vi "GetReferenceByUID_traverser.vi"(4 "context in":variant, 5 "objref":refnum<vi>) -> (1 "context out":variant, 2 "traverse flags":i32)   [LabVIEW 2013]
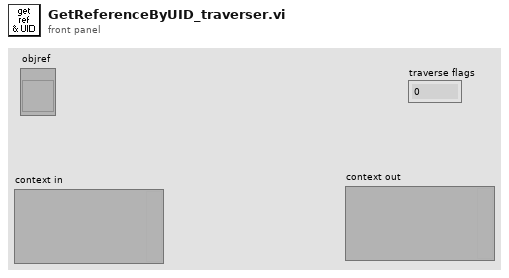
[diagram p1: front panel]
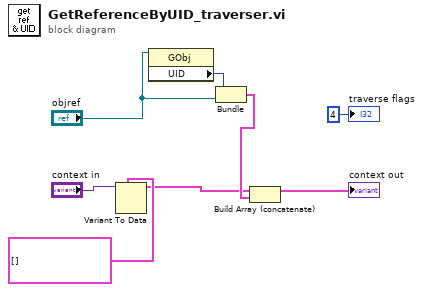
[diagram p0: block diagram]
diagram:
  n1 = Variant To Data(type=cluster{"UID":i32, "objref":refnum<vi>}[] [] ("appended array"), Variant="context in") -> (data=w1:cluster{"UID":i32, "objref":refnum<vi>}[])  [unwired: 1 in, 1 out]
  n2 = property class="GObj"(reference="objref") -> ("UID"=w5:i32)  [unwired: 1 in, 2 out]
  n3 = Bundle("UID"=w5, "objref"="objref") -> (w3:cluster{"UID":i32, "objref":refnum<vi>})  [unwired: 1 in]
  n4 = Build Array (concatenate)(w1, w3) -> (→"context out":cluster{"UID":i32, "objref":refnum<vi>}[])
  "traverse flags" <- 4 ("Traverse Flags")
